vi "Read Steps State.vi"(8 "error in (no error)":errorcluster, 11 "Parallel Step in":refnum<class "Parallel Step.lvclass">) -> (0 "error out":errorcluster, 2 "Steps State":T1[](array[typedef]), 3 "Parallel Step out":refnum<class "Parallel Step.lvclass">)   [LabVIEW 2015, in "Parallel Step.lvclass"]
uses:
  Parallel Step.lvclass
  classes/Step/Execution/StepState.ctl
  classes/Step/Execution/Step Status.ctl
  classes/Step/Execution/Step Flow Control.ctl
  Parallel Step.lvclass/Parallel Step.ctl
  classes/Step/Execution/Step.lvclass
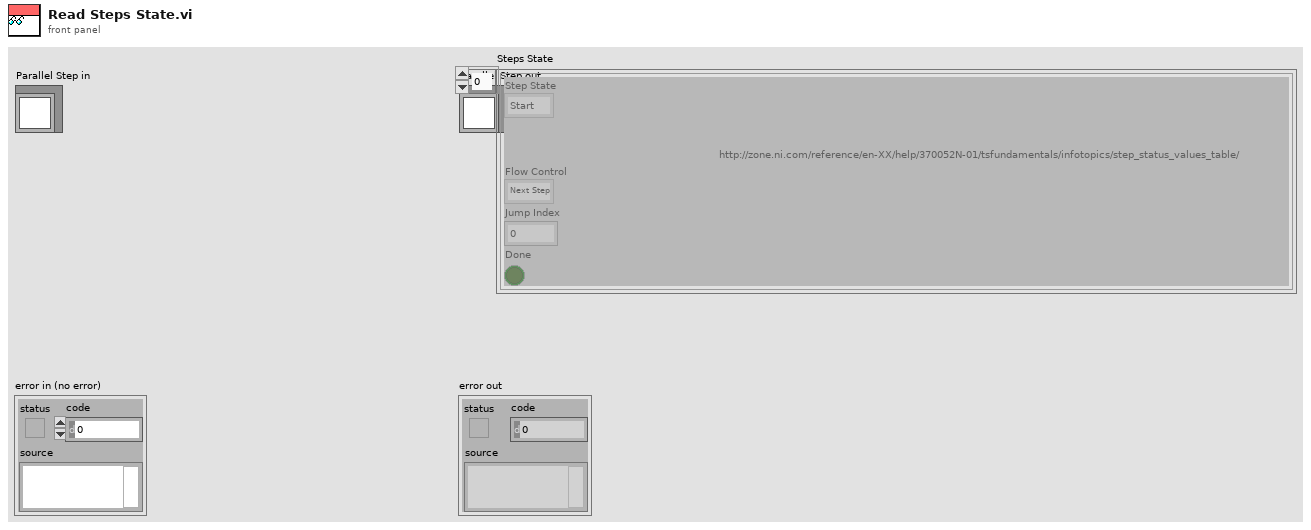
[diagram p1: front panel]
types:
  T1 = typedef "Step.lvclass/StepState.ctl" = cluster{"Step State":T2, "Flow Control":T3, "Jump Index":i32, "Done":bool}
  T2 = typedef "Step.lvclass/Step Status.ctl" = enum16{"Start", "Passed", "Failed", "Error", "Done", "Terminated", "Skipped", "Running"}
  T3 = typedef "Step.lvclass/Step Flow Control.ctl" = enum16{"Next Step", "Jump"}
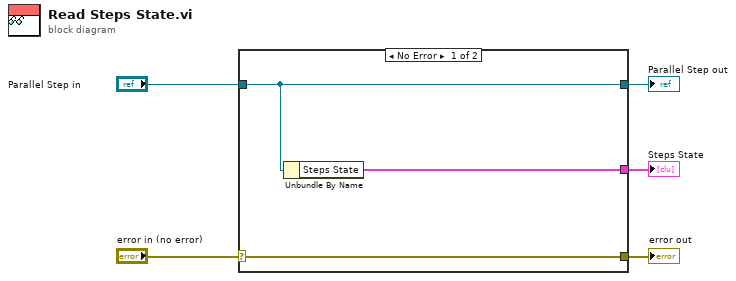
[diagram p0: block diagram]
diagram:
  n1 = case shown="No Error" "error in (no error)" {
    selector: "error in (no error)" -> [w8 w9]
    tunnel: [w8 w9] -> w4
    tunnel: [w7 w10] -> w2
    tunnel: "Parallel Step in" -> [w7 w10]
    tunnel: [w6 _] -> w1
    frame No Error {
      n2 = Unbundle By Name(w7) -> ("Steps State"=w6:T1[])
    }
    frame Error {
    }
  }
  "error out" <- w4
  "Parallel Step out" <- w2
  "Steps State" <- w1
